vi "串口控制PLC.vi"() -> ()   [LabVIEW 2018]
uses:
  <vilib>/Instr/_visa.llb/VISA Configure Serial Port (Instr).vi
panel:
  in  "断开指令":string
  in  "控制":bool
  out "错误输出":errorcluster
  in  "read（T）":bool
  in  "Delay Time (s)":dbl=1.0 caption="延迟时间(s)"
  in  "延迟500ms":u32=500
  out "返回数":u32
  in  "吸合指令":string
  in  "stop bits (10: 1 bit)":u16(ring)=10 items=["1.0"=10, "1.5"=15, "2.0"=20]
  in  "parity (0:none)":enum16{"None", "Odd", "Even", "Mark", "Space"}(ring)
  in  "data bits (8)":u16=8 min=5 max=8 step=1
  in  "baud rate (9600)":u32=9600
  in  "请选择串口号":refnum<visa-resource-name>
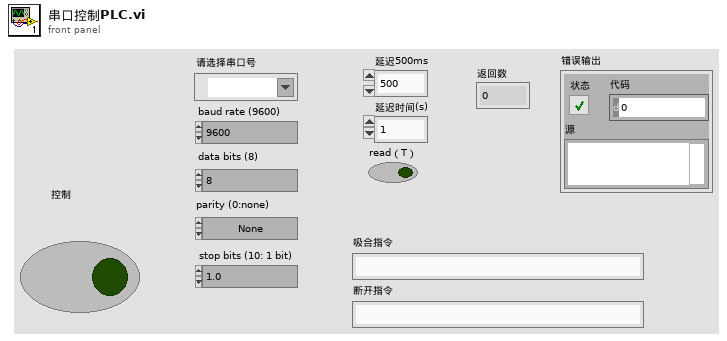
[diagram p1: front panel]
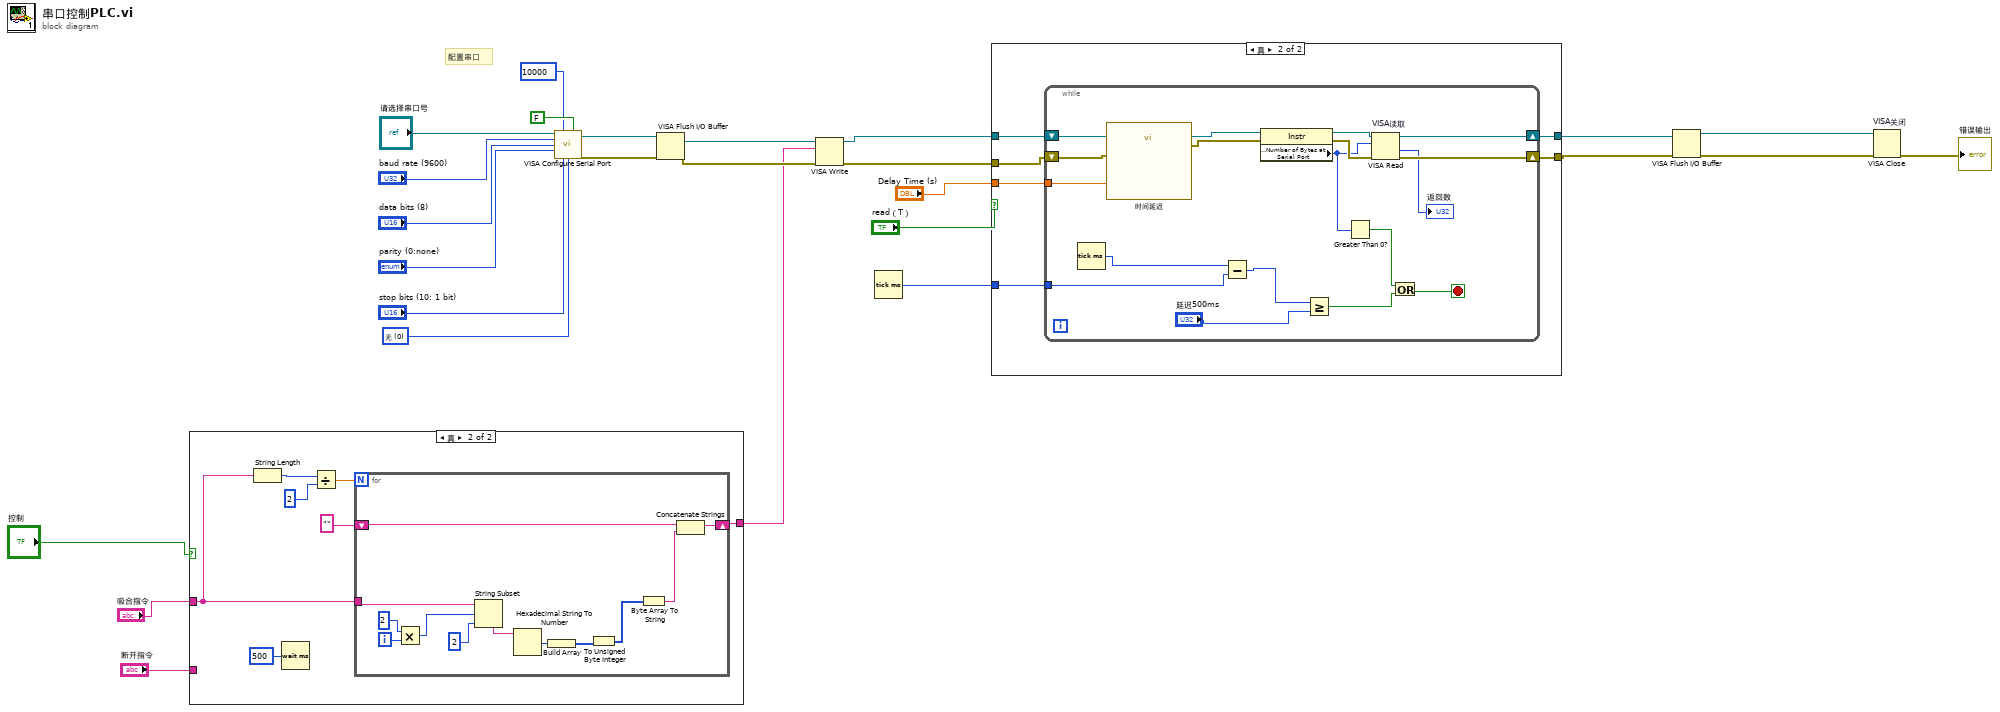
[diagram p0: block diagram]
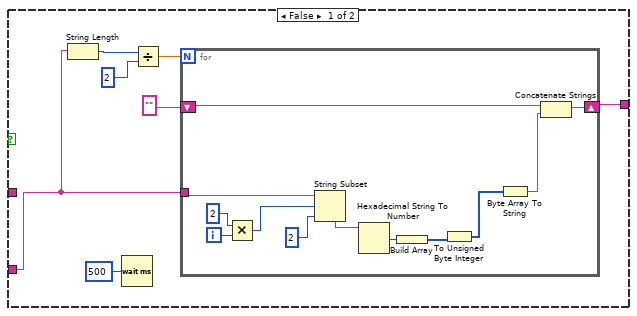
[diagram p2: hidden frame]
diagram:
  w16 = u16 0 items=["无", "XON/XOFF", "RTS/CTS", "XON/XOFF & RTS/CTS", "DTR/DSR", "XON/XOFF & DTR/DSR"] ("flow control (0:none)")
  # "配置串口"
  n1 = case shown="真" "控制" {
    tunnel: [w29 w48] -> w5
    tunnel: "断开指令" -> [w27 _]
    tunnel: "吸合指令" -> [_ w46]
    frame False {
      n2 = String Length(string=w27) -> (length=w32:i32)
      n3 = Wait (ms)(milliseconds to wait=u32 500 ("等待时间（毫秒）")) -> ()  [unwired: 1 out]
      n4 = Divide(x=w32, y=2) -> (x/y=w31:dbl)
      n5 = for {
        N: w31 -> [_]
        tunnel: w27 -> [w37]
        shift-right: [w42] -> w29
        shift-left: "" -> [w38]
        i -> [w45]
        n6 = Multiply(x=2, y=w45) -> (x*y=w35:i32)
        n7 = String Subset(string=w37, offset (0)=w35, length (rest)=2 ("长度（子字符串长度）")) -> (substring=w36:string)
        n8 = Hexadecimal String To Number(string=w36) -> (number=w40:u32)  [unwired: 2 in, 1 out]
        n9 = Build Array(w40) -> (w39:u32[])
        n10 = To Unsigned Byte Integer(number=w39) -> (unsigned 8bit integer=w41:u8[])
        n11 = Byte Array To String(unsigned byte array=w41) -> (string=w43:string)
        n12 = Concatenate Strings(w38, w43) -> (w42:string)
      }
    }
    frame True {
      n13 = String Length(string=w46) -> (length=w51:i32)
      n14 = Wait (ms)(milliseconds to wait=u32 500 ("等待时间（毫秒）")) -> ()  [unwired: 1 out]
      n15 = Divide(x=w51, y=2) -> (x/y=w50:dbl)
      n16 = for {
        N: w50 -> [_]
        tunnel: w46 -> [w56]
        shift-right: [w61] -> w48
        shift-left: "" -> [w57]
        i -> [w64]
        n17 = Multiply(x=2, y=w64) -> (x*y=w54:i32)
        n18 = String Subset(string=w56, offset (0)=w54, length (rest)=2 ("长度（子字符串长度）")) -> (substring=w55:string)
        n19 = Hexadecimal String To Number(string=w55) -> (number=w59:u32)  [unwired: 2 in, 1 out]
        n20 = Build Array(w59) -> (w58:u32[])
        n21 = To Unsigned Byte Integer(number=w58) -> (unsigned 8bit integer=w60:u8[])
        n22 = Byte Array To String(unsigned byte array=w60) -> (string=w62:string)
        n23 = Concatenate Strings(w57, w62) -> (w61:string)
      }
    }
  }
  n24 = call-poly "VISA Configure Serial Port"("VISA resource name"="请选择串口号", "timeout (10sec)"=u32 10000, "Enable Termination\nChar (T)"=FALSE ("Enable Termination\nChar (T)"), "baud rate (9600)"="baud rate (9600)", "data bits (8)"="data bits (8)", "parity (0:none)"="parity (0:none)", "stop bits (10: 1 bit)"="stop bits (10: 1 bit)", "flow control (0:none)"=w16) -> ("VISA resource name out"=w20:refnum<visa-resource-name>, "error out"=w19:errorcluster)  [unwired: 6 in]
  n25 = VISA Flush I/O Buffer(VISA resource name=w20, error in (no error)=w19) -> (VISA resource name out=w18:refnum<visa-resource-name>, error out=w17:errorcluster)  [unwired: 1 in]
  n26 = VISA Write(VISA resource name=w18, write buffer=w5, error in (no error)=w17) -> (VISA resource name out=w13:refnum<visa-resource-name>, error out=w14:errorcluster)  [unwired: 1 out]
  n27 = Tick Count (ms)() -> (millisecond timer value=w12:u32)
  n28 = case shown="真" "read（T）" {
    tunnel: [w66 w72] -> w9
    tunnel: [w65 w71] -> w8
    tunnel: w14 -> [w65 w70]
    tunnel: w13 -> [w66 w69]
    tunnel: w12 -> [_ w68]
    tunnel: "Delay Time (s)" -> [_ w67]
    frame False {
    }
    frame True {
      n29 = while {
        tunnel: w68 -> [w80]
        shift-right: [w86] -> w71
        shift-left: w70 -> [w84]
        shift-right: [w87] -> w72
        shift-left: w69 -> [w83]
        tunnel: w67 -> [w73]
        stop <- w76 stop-if-true
        n30 = Tick Count (ms)() -> (millisecond timer value=w81:u32)
        n31 = call "时间延迟"("error in (no error)"=w84, "Delay Time (s)"=w73) -> ("error out"=w85:errorcluster)  [unwired: 9 in]
        n32 = Subtract(x=w81, y=w80) -> (x-y=w79:u32)
        n33 = property class="Instr"(reference=w83, error in=w85) -> (reference out=w89:refnum<visa-resource-name>, error out=w88:errorcluster, "Serial Settings:Number of Bytes at Serial Port"=w75:u32)
        n34 = Greater Or Equal?(x=w79, y="延迟500ms") -> (x >= y?=w77:bool)
        n35 = Greater Than 0?(x=w75) -> (x > 0?=w78:bool)
        n36 = VISA Read "VISA读取"(VISA resource name=w89, byte count=w75, error in (no error)=w88) -> (VISA resource name out=w87:refnum<visa-resource-name>, return count=→"返回数":u32, error out=w86:errorcluster)  [unwired: 1 out]
        n37 = Or(x=w78, y=w77) -> (x .or. y?=w76:bool)
      }
    }
  }
  n38 = VISA Flush I/O Buffer(VISA resource name=w9, error in (no error)=w8) -> (VISA resource name out=w7:refnum<visa-resource-name>, error out=w6:errorcluster)  [unwired: 1 in]
  n39 = VISA Close "VISA关闭"(VISA resource name=w7, error in (no error)=w6) -> (error out=→"错误输出":errorcluster)
